vi "convert float.vi"(10 "Numeric":dbl) -> (2 "result string":string)   [LabVIEW 2026]
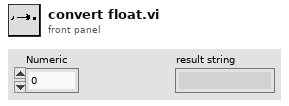
[diagram p1: front panel]
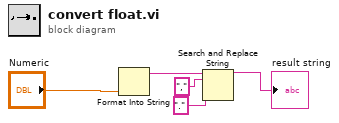
[diagram p0: block diagram]
diagram:
  n1 = Format Into String("Numeric") -> (resulting string=w4:string)  [unwired: 3 in, 1 out]
  n2 = Search and Replace String(input string=w4, search string=",", replace string="." ("replace string (\"\")")) -> (result string=→"result string":string)  [unwired: 5 in, 3 out]
